vi "Create Internal Stop Enqueuer.vi"(8 "error in (no error)":errorcluster) -> (0 "error out":errorcluster, 2 "Stop Enqueuer":refnum<user-event>, 3 "Internal-Stop":refnum<event-registration>)   [LabVIEW 2018, in "Scripting.lvlib" / "Actor.lvclass"]
uses:
  Actor.lvclass
  Internal-Stop.ctl
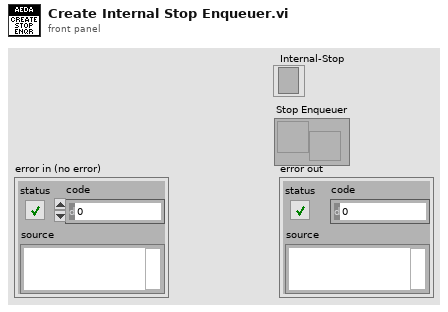
[diagram p1: front panel]
types:
  T1 = typedef "Scripting.lvlib/Actor.lvclass/Internal-Stop.ctl" = cluster{"Type":enum16{"Normal", "Emergency"}}
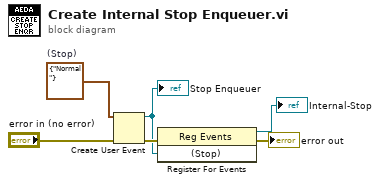
[diagram p0: block diagram]
diagram:
  w6 = T1 {"Type"=enum."Normal"}  # (Stop)
  n1 = Create User Event(user event datatype=w6, error in="error in (no error)") -> (user event=w2:refnum<user-event>, error out=w4:errorcluster)
  "Stop Enqueuer" <- w2
  n2 = register-events(error in=w4, w2) -> (reference out=→"Internal-Stop":refnum<event-registration>, error out=→"error out":errorcluster)  [unwired: 1 in]
